vi "FilesCount.vi"(0 "NomProjet":string, 1 "entrée d'erreur":errorcluster) -> (2 "cheminProchainFichierTDMS":path, 3 "NomProchainFichier":string, 4 "noms des fichiers":string[](array[string]), 5 "cheminProchainFichierValise":path, 6 "NextTestNum":u32, 7 "sortie d'erreur":errorcluster)   [LabVIEW 2017]
doc: "Ce VI renvoie le nombre de fichier de mesures présents dans le repertoire du projet en cours"
uses:
  DefDeType/WhichPath.ctl
panel:
  out "longueur":i32
  out "Tableau 2":i32[](array[numeric])
  out "Tableau":string[](array[string])
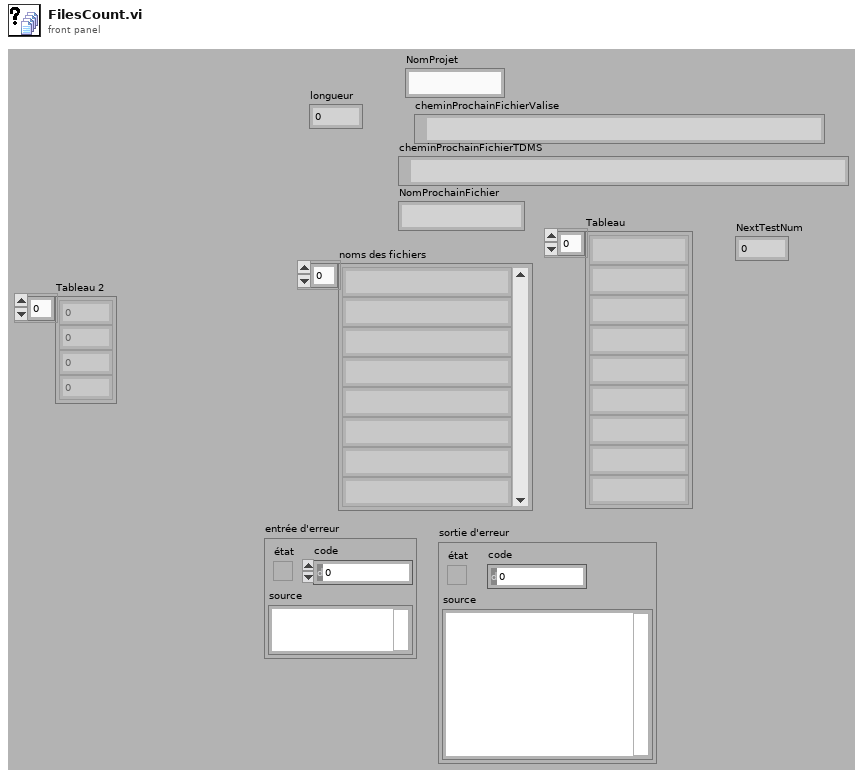
[diagram p1: front panel]
types:
  T1 = typedef "WhichPath.ctl" = enum16{"DossierProjet", "Config", "Meas", "MeasPCI", "MeasCRIO1", "MeasCRIO2", "MeasQualisys", "MeasHBM", "MeasTDMS", "Fig", "Res"}
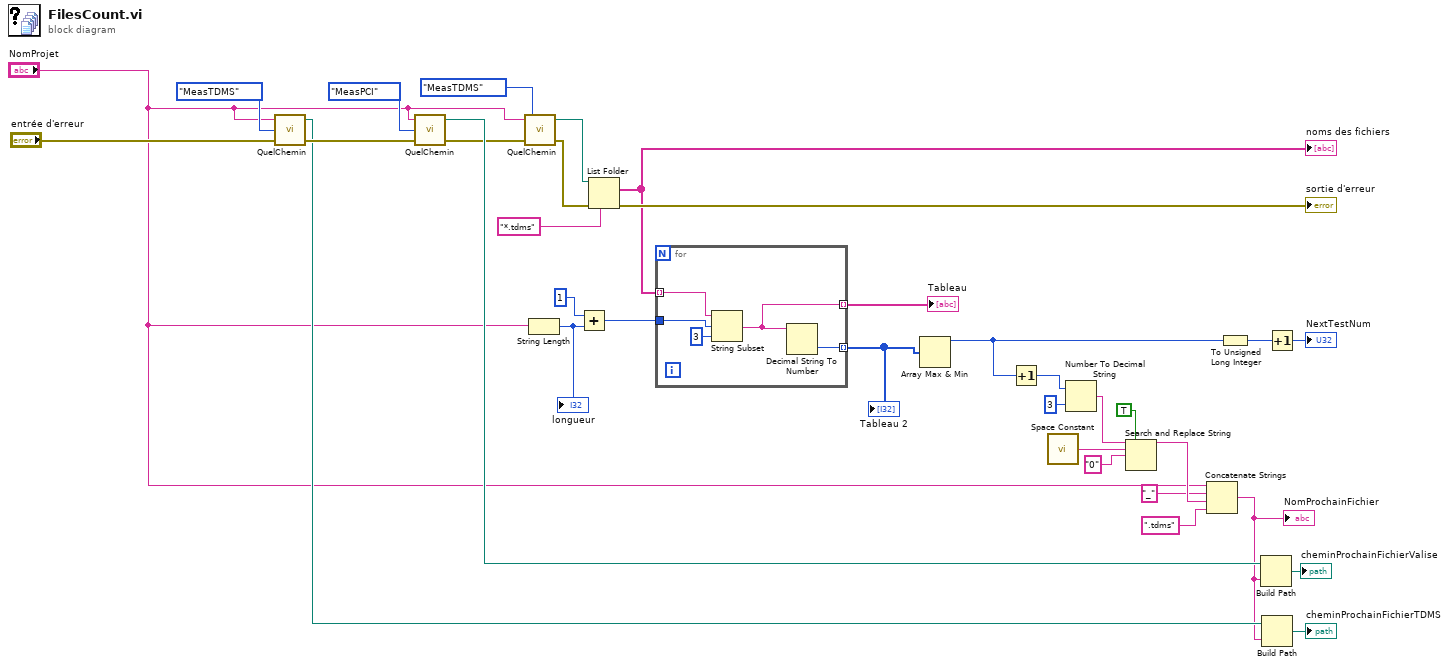
[diagram p0: block diagram]
diagram:
  n1 = call "QuelChemin.vi"("Entrée d'erreur"="entrée d'erreur", "WhichPath?"=WhichPath."MeasTDMS", "NomProjet"="NomProjet") -> ("Sortie d'erreur"=w13:errorcluster, "SurDisqueLocal"=w11:path)  [unwired: 1 out]
  n2 = call "QuelChemin.vi"("Entrée d'erreur"=w13, "WhichPath?"=WhichPath."MeasPCI", "NomProjet"="NomProjet") -> ("Sortie d'erreur"=w8:errorcluster, "SurDisqueLocal"=w16:path)  [unwired: 1 out]
  n3 = call "QuelChemin.vi"("Entrée d'erreur"=w8, "WhichPath?"=WhichPath."MeasTDMS", "NomProjet"="NomProjet") -> ("Sortie d'erreur"=w7:errorcluster, "SurDisqueLocal"=w4:path)  [unwired: 1 out]
  n4 = String Length(string="NomProjet") -> (length=w31:i32)
  "longueur" <- w31
  n5 = Add(x=1, y=w31) -> (x+y=w33:i32)
  n6 = List Folder(path=w4, pattern="*.tdms" ("chaîne"), error in=w7) -> (filenames=w28:string[], error out=→"sortie d'erreur":errorcluster)  [unwired: 3 out]
  "noms des fichiers" <- w28
  n7 = for {
    tunnel: w28 -> [w37] mode=indexing
    tunnel: w33 -> [w39]
    tunnel: [w36] -> w32 mode=indexing
    tunnel: [w35] -> w30 mode=indexing
    n8 = String Subset(string=w37, offset (0)=w39, length (rest)=3 ("longueur (reste)")) -> (substring=w35:string)
    n9 = Decimal String To Number(string=w35) -> (number=w36:i32)  [unwired: 3 out]
  }
  "Tableau" <- w30
  "Tableau 2" <- w32
  n10 = Array Max & Min(array=w32) -> (max value=w26:i32)  [unwired: 3 out]
  n11 = Increment(x=w26) -> (x+1=w25:i32)
  n12 = call <vilib>:"Space Constant.vi"() -> ("String"=w22:string)
  n13 = Number To Decimal String(number=w25, width (-)=i16 3 ("largeur (-)")) -> (decimal integer string=w23:string)
  n14 = Search and Replace String(replace all?=TRUE ("tout remplacer ? (F)"), input string=w23, search string=w22, replace string="0" ("chaîne de remplacement (\"\")")) -> (result string=w20:string)  [unwired: 4 in, 3 out]
  n15 = Concatenate Strings("NomProjet", "_" ("chaîne"), w20, ".tdms" ("chaîne")) -> (w10:string)
  "NomProchainFichier" <- w10
  n16 = To Unsigned Long Integer(number=w26) -> (unsigned 32bit integer=w2:u32)
  n17 = Build Path(base path=w16, name or relative path=w10) -> (appended path=→"cheminProchainFichierValise":path)
  n18 = Build Path(base path=w11, name or relative path=w10) -> (appended path=→"cheminProchainFichierTDMS":path)
  n19 = Increment(x=w2) -> (x+1=→"NextTestNum":u32)
